vi "Enforce Pulse Range.vi"(8 "error in":errorcluster, 10 "Ideal Range":cluster{"Low":dbl, "High":dbl}, 11 "3300 in":refnum<class "3300.lvclass">) -> (0 "error out":errorcluster, 3 "3300 out":refnum<class "3300.lvclass">)   [LabVIEW 2019, in "3300.lvlib" / "3300.lvclass"]
uses:
  Library/3300.lvclass
  C:/Users/Public/Documents/Development/builds/Instruments/Electronic Load.lvlibp/Library/Electronic Load.lvclass
  builds/Instruments/Electronic Load.lvlibp/Private/GUI/Read Trigger_Ref.vi
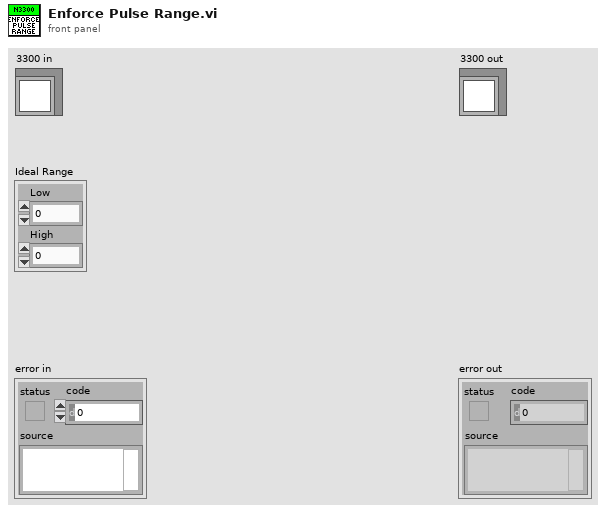
[diagram p1: front panel]
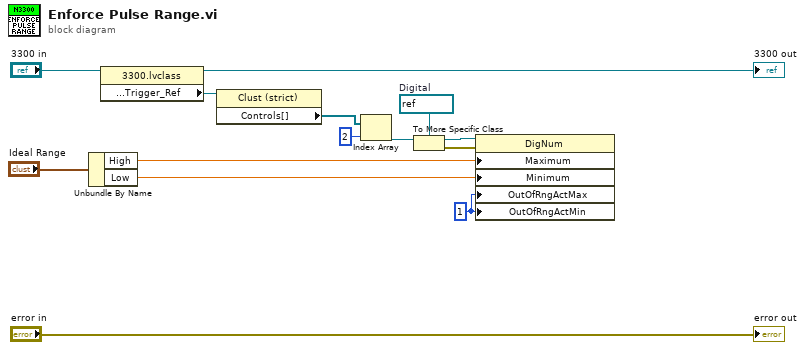
[diagram p0: block diagram]
diagram:
  w6 = u8 1 ("Response to Value Outside Limits:Minimum")
  w9 = refnum<vi> refnum  # Digital
  n1 = Unbundle By Name("Ideal Range") -> ("High"=w4:dbl, "Low"=w3:dbl)
  n2 = property class="3300.lvclass"(reference="3300 in") -> (reference out=→"3300 out":refnum<class "3300.lvclass">, "Protected:Accessors:GUI:Trigger_Ref"=w13:refnum<vi>)  [unwired: 1 in, 1 out]
  n3 = property class="Clust (strict)"(reference=w13) -> ("Controls[]"=w12:refnum<vi>[])  [unwired: 1 in, 2 out]
  n4 = Index Array(array=w12, index=2) -> (element=w10:refnum<vi>)
  n5 = To More Specific Class(target class=w9, reference=w10) -> (specific class reference=w8:refnum<vi>, error out=w7:errorcluster)  [unwired: 1 in]
  n6 = property class="DigNum"(reference=w8, error in=w7, "Maximum"=w4, "Minimum"=w3, "OutOfRngActMax"=w6, "OutOfRngActMin"=w6) -> ()  [unwired: 2 out]
  "error out" <- "error in"
